vi "T11 - Усреднение напряжений по нескольким отсчетам АЦП.vi"() -> ()   [LabVIEW 2009]
uses:
  Z210/Z210 CTL Lib.llb/Z210 CTL ADC Voltages.ctl
  Z210/Z210 CTL Lib.llb/Z210 CTL ADC or DAC Function.ctl
  Instance          15 62Saved   T11 - Усреднение напряжений по нескольким отсчетам АЦП .vi
  Instance          16 62Saved   T11 - Усреднение напряжений по нескольким отсчетам АЦП .vi
  Instance          17 62Saved   T11 - Усреднение напряжений по нескольким отсчетам АЦП .vi
  Instance          18 62Saved   T11 - Усреднение напряжений по нескольким отсчетам АЦП .vi
  Instance          19 62Saved   T11 - Усреднение напряжений по нескольким отсчетам АЦП .vi
  Instance          20 62Saved   T11 - Усреднение напряжений по нескольким отсчетам АЦП .vi
  Instance          21 62Saved   T11 - Усреднение напряжений по нескольким отсчетам АЦП .vi
  Instance          22 62Saved   T11 - Усреднение напряжений по нескольким отсчетам АЦП .vi
  Instance          23 62Saved   T11 - Усреднение напряжений по нескольким отсчетам АЦП .vi
  <vilib>/Analysis/NI_AALBase.lvlib
panel:
  out "max value":dbl
  in  "Усреднить по":i32=1
  out "Стд. отклонение напряжения":cluster{"Y":dbl[], "Y":dbl[]}[](graph)
  out "ADC StdDevs'":dbl[unit][](array[numeric])
  out "Число циклов ожидания пакета":cluster{"Y":dbl[], "Y":dbl[]}[](graph)
  out "Время отклика":cluster{"Y":dbl[], "Y":dbl[]}[](graph)
  in  "stop":bool
  in  "Напряжение ЦАП_1":dbl[unit]=1.0
  out "Напряжения АЦП":T1
  in  "ADC freq":dbl[unit]
  out "DAC buffer size":i32=32768
  # "Позволяет управлять величиной постоянного напряжения, генерируемого первым (нулевым, если следовать\nнумерации) каналом ЦАП. И регистрировать это напряжение, подведенное к первому каналу АЦП, включенному\nв синфазном режиме. Гистограмма Время отклика позволяет оценить сколько времени проходит от установки\nнапряжения ЦАП до считывания значения напряжения АЦП. Гистограмма Число циклов ожидания пакета дает \nпредставление о том, как часто приходят пакеты данных АЦП, при выбранной частоте дискретизации. \nГистограмма Стд. отклонение напряжения дает представление о характерном масштабе погрешности при измерении\nнапряжения."
  # "1. Соединить землю АЦП и ЦАП\n2. Соединить вывод 1 ЦАП и вывод 1 АЦП\n3. Запустить\n4а. Изменить число отсчетов, по которому следует проводить усреднение. Убедиться что при \n•  10 отсчетах погрешность не более 1E-3 время отклика в пределах 6-10 мс.\n•  3000 отсчетов погрешность не более 6E-4 время отклика в пределах 6-10 мс.\n4б. При неразумном числе отсчетов (очень большом или 0) получи ошибку."
  # "отсчетам"
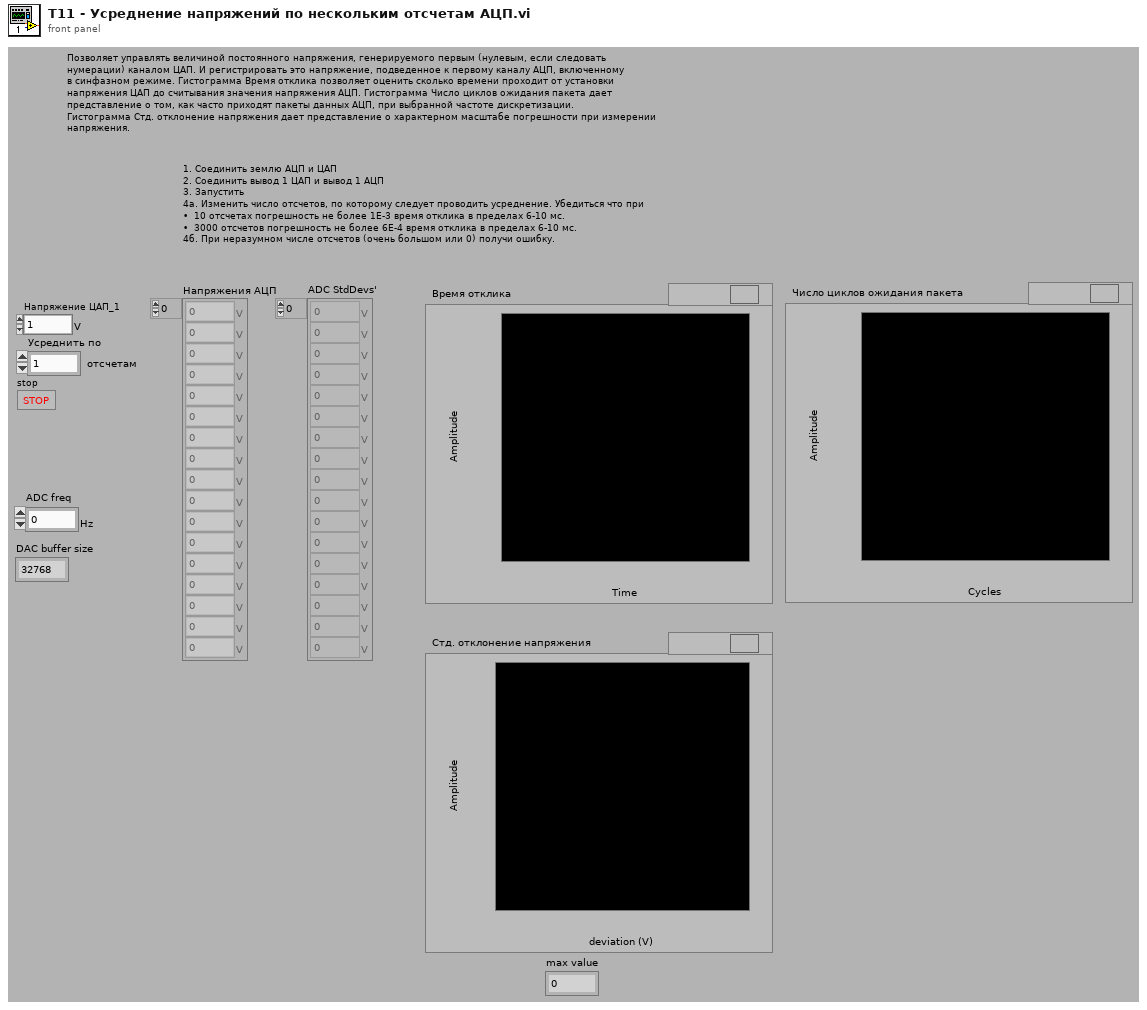
[diagram p1: front panel]
types:
  T1 = typedef "Z210 CTL ADC Voltages.ctl" = dbl[unit][]
  T2 = typedef "Z210 CTL ADC or DAC Function.ctl" = enum16{"АЦП", "ЦАП", "Both"}
  T3 = typedef "Z210 CTL Unit Data .ctl" = cluster{"typeDevice":i32, "numberDSP":i32}
  T4 = typedef "Z210 CTL Buffers Params.ctl" = cluster{"bufferAddr ADC":u32, "bufferSize ADC":i32, "bufferAddr DAC":u32, "bufferSize DAC":i32}
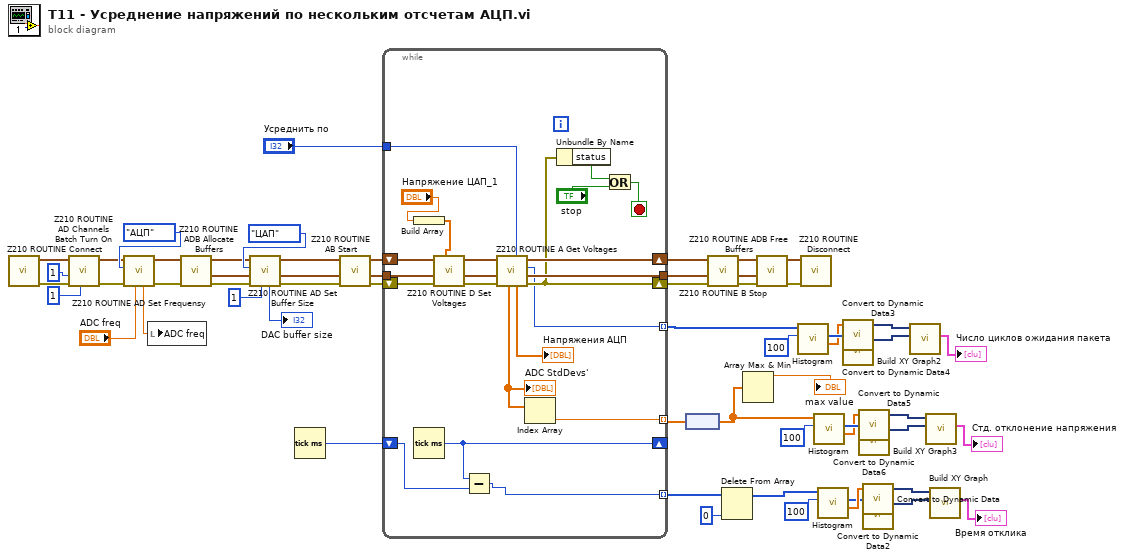
[diagram p0: block diagram]
diagram:
  n1 = call "Z210 ROUTINE Connect.vi"() -> ("error out"=w57:errorcluster, "unitData out"=w58:T3)  [unwired: 10 in]
  n2 = call "Z210 ROUTINE AD Channels Batch Turn On.vi"("N ЦАП (0)"=1, "error in (no error)"=w57, "N Синф (0)"=1, "unitData in"=w58) -> ("error out"=w35:errorcluster, "unitData out"=w36:T3)  [unwired: 4 in, 2 out]
  n3 = call "Z210 ROUTINE AD Set Frequensy.vi"("freq suggestion"="ADC freq", "error in (no error)"=w35, "AorD"=Z210_CTL_ADC_or_DAC_Function."АЦП", "unitData in"=w36) -> ("error out"=w33:errorcluster, "unitData out"=w34:T3, "freq"=w49:dbl[unit])  [unwired: 5 in]
  n4 = local write "ADC freq"(w49) -> ()
  n5 = call "Z210 ROUTINE ADB Allocate Buffers.vi"("error in (no error)"=w33, "unitData in"=w34) -> ("error out"=w31:errorcluster, "buffersParams out"=w30:T4, "unitData out"=w32:T3)  [unwired: 7 in]
  n6 = call "Z210 ROUTINE AD Set Buffer Size.vi"("size suggestion (0)"=1, "error in (no error)"=w31, "buffersParams"=w30, "AorD"=Z210_CTL_ADC_or_DAC_Function."ЦАП", "unitData in"=w32) -> ("error out"=w47:errorcluster, "buffersParams out"=w46:T4, "unitData out"=w48:T3, "size"=→"DAC buffer size":i32)  [unwired: 3 in]
  n7 = Tick Count (ms)() -> (millisecond timer value=w29:u32)
  n8 = call "Z210 ROUTINE AB Start.vi"("error in (no error)"=w47, "buffersParams"=w46, "unitData in"=w48) -> ("error out"=w45:errorcluster, "buffersParams out"=w43:T4, "unitData out"=w44:T3)  [unwired: 6 in]
  n9 = while {
    tunnel: w43 -> [w76]
    shift-right: [w70] -> w41
    shift-left: w45 -> [w80]
    shift-right: [w74] -> w42
    shift-left: w44 -> [w79]
    tunnel: [w73] -> w12
    shift-right: [w66] -> _
    shift-left: w29 -> [w67]
    tunnel: [w65] -> w22 mode=indexing
    tunnel: [w62] -> w13 mode=indexing
    tunnel: [w60] -> w10 mode=indexing
    tunnel: "Усреднить по" -> [w59]
    stop <- w69 stop-if-true
    n10 = Build Array("Напряжение ЦАП_1") -> (w63:dbl[unit][])
    n11 = Tick Count (ms)() -> (millisecond timer value=w66:u32)
    n12 = call "Z210 ROUTINE D Set Voltages.vi"("DAC Voltages"=w63, "error in (no error)"=w80, "buffersParams"=w76, "unitData in"=w79) -> ("error out"=w77:errorcluster, "buffersParams out"=w75:T4, "unitData out"=w78:T3)  [unwired: 5 in]
    n13 = Subtract(x=w66, y=w67) -> (x-y=w65:u32)
    n14 = call "Z210 ROUTINE A Get Voltages.vi"("N to average (1)"=w59, "error in (no error)"=w77, "buffersParams"=w75, "unitData in"=w78) -> ("error out"=w70:errorcluster, "buffersParams out"=w73:T4, "cyclesWaited"=w62:i32, "unitData out"=w74:T3, "ADC Voltages"=→"Напряжения АЦП":T1, "ADC StdDevs'"=w61:dbl[unit][])  [unwired: 2 in]
    "ADC StdDevs'" <- w61
    n15 = Index Array(array=w61) -> (element=w60:dbl[unit])  [unwired: 1 in]
    n16 = Unbundle By Name(w70) -> ("status"=w68:bool)
    n17 = Or(x=w68, y="stop") -> (x .or. y?=w69:bool)
  }
  n18 = node(w10) -> (w2:dbl[])
  n19 = call "Z210 ROUTINE B Stop.vi"("error in (no error)"=w41, "buffersParams"=w12, "unitData in"=w42) -> ("error out"=w39:errorcluster, "buffersParams out"=w11:T4, "unitData out"=w40:T3)  [unwired: 6 in]
  n20 = Delete From Array(array=w22, index=0) -> (array with subset deleted=w21:u32[])  [unwired: 1 in, 1 out]
  n21 = Array Max & Min(array=w2) -> (max value=→"max value":dbl)  [unwired: 3 out]
  n22 = call "Z210 ROUTINE ADB Free Buffers.vi"("error in (no error)"=w39, "buffersParams"=w11, "unitData in"=w40) -> ("error out"=w37:errorcluster, "unitData out"=w38:T3)  [unwired: 6 in, 1 out]
  n23 = call <vilib>:"Histogram.vi"("intervals"=100, "X"=w13) -> ("X Values"=w16:dbl[], "Histogram: h(x)"=w18:i32[])  [unwired: 6 in, 2 out]
  n24 = call "Z210 ROUTINE Disconnect.vi"("error in (no error)"=w37, "unitData in"=w38) -> ()  [unwired: 8 in, 2 out]
  n25 = call <vilib>:"Histogram.vi"("intervals"=100, "X"=w2) -> ("X Values"=w6:dbl[], "Histogram: h(x)"=w8:i32[])  [unwired: 6 in, 2 out]
  n26 = call <vilib>:"Histogram.vi"("intervals"=100, "X"=w21) -> ("X Values"=w26:dbl[], "Histogram: h(x)"=w24:i32[])  [unwired: 6 in, 2 out]
  n27 = call "Convert to Dynamic Data3"("Array"=w16) -> ("Dynamic Data Type"=w17:dynamicdata)  [unwired: 3 in]
  n28 = call "Convert to Dynamic Data4"("Array"=w18) -> ("Dynamic Data Type"=w19:dynamicdata)  [unwired: 3 in]
  n29 = call "Convert to Dynamic Data5"("Array"=w6) -> ("Dynamic Data Type"=w7:dynamicdata)  [unwired: 3 in]
  n30 = call "Convert to Dynamic Data6"("Array"=w8) -> ("Dynamic Data Type"=w9:dynamicdata)  [unwired: 3 in]
  n31 = call "Convert to Dynamic Data"("Array"=w26) -> ("Dynamic Data Type"=w25:dynamicdata)  [unwired: 3 in]
  n32 = call "Convert to Dynamic Data2"("Array"=w24) -> ("Dynamic Data Type"=w23:dynamicdata)  [unwired: 3 in]
  n33 = call "Build XY Graph2"("Y Input"=w19, "X Input"=w17) -> ("XY Graph"=→"Число циклов ожидания пакета":cluster{"Y":dbl[], "Y":dbl[]}[])  [unwired: 8 in, 1 out]
  n34 = call "Build XY Graph3"("Y Input"=w9, "X Input"=w7) -> ("XY Graph"=→"Стд. отклонение напряжения":cluster{"Y":dbl[], "Y":dbl[]}[])  [unwired: 8 in, 1 out]
  n35 = call "Build XY Graph"("Y Input"=w23, "X Input"=w25) -> ("XY Graph"=→"Время отклика":cluster{"Y":dbl[], "Y":dbl[]}[])  [unwired: 8 in, 1 out]
